vi "convert temperature back to thermocouple voltage.vi"(3 "CJC R_T":sgl, 4 "ThermocoupleType":u16(ring)=6 items=["B", "E", "J", "K", "R", "S", "T", "N"], 5 "Temperature (K)":sgl format="%0.6f") -> (1 "thermocouple voltage signal":sgl)   [LabVIEW 2018]
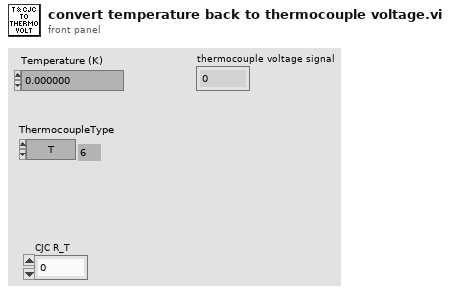
[diagram p1: front panel]
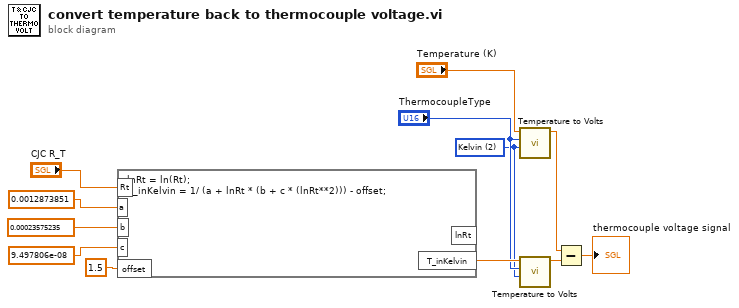
[diagram p0: block diagram]
diagram:
  w3 = u16 2 items=["Celsius", "Fahrenheit", "Kelvin", "Rankine"] ("Temperature Units")
  n1 = formula code="lnRt = ln(Rt);\nT_inKelvin = 1/ (a + lnRt * (b + c * (lnRt**2))) - offset;"("a"=0.0012873851, "b"=0.00023575235, "c"=9.497806e-08, "Rt"="CJC R_T", "offset"=1.5 ("input variable")) -> ("T_inKelvin"=w5:dbl)  [unwired: 1 out]
  n2 = call <vilib>:"Temperature to Volts.vi"("Temperature Units"=w3, "ThermocoupleType"="ThermocoupleType", "Temperature"="Temperature (K)") -> ("Thermocouple Voltage"=w6:sgl)  [unwired: 4 in]
  n3 = call <vilib>:"Temperature to Volts.vi"("Temperature Units"=w3, "ThermocoupleType"="ThermocoupleType", "Temperature"=w5) -> ("Thermocouple Voltage"=w2:sgl)  [unwired: 4 in]
  n4 = Subtract(x=w6, y=w2) -> (x-y=→"thermocouple voltage signal":sgl)
